vi "imp_2motor_v1.vi"() -> ()   [LabVIEW 2014]
uses:
  <vilib>/LabVIEW Targets/FPGA/cRIO/shared/nicrio_ModuleControls/nicrio_cRIO-9237_DataRatesRing.ctl
  <vilib>/LabVIEW Targets/FPGA/cRIO/shared/nicrio_ModuleControls/nicrio_cRIO-9237_ExcitationVoltageRing.ctl
  <vilib>/rvi/FXPMathLib/FxpSinAndCos/subVIs/nifxpmath_SinAndCos_SimConfig.ctl
  <vilib>/rvi/Emulation/niFpgaGetClockAttributes.vi
  <vilib>/rvi/Emulation/niFpgaSctlEmulationGetInTimedLoop.vi
  <vilib>/rvi/Emulation/niFpgaEmulationReportErrorSimple.vi
  <vilib>/rvi/Emulation/niFpgaProcessEmulError.vi
  <vilib>/rvi/interface/RandomDataEmulation/nirviRandomDataMultiElementFPGAFIFO.vi
  <instcachedir>/0/nirviRandomDataMultiElementFPGAFIFO_AD0CFC12EF974623A9C2E4184BC062B2.lvgen/nirviRandomDataMultiElementFPGAFIFO_AD0CFC12EF974623A9C2E4184BC062B2_023.vi
  <vilib>/rvi/interface/RandomDataEmulation/niFpgaRandomDataHandleErrors.vi
  <vilib>/rvi/Emulation/niFpgaCriticalErrorInLSC.vi
  <vilib>/rvi/eio/common/nirviEmuTemplateMethod_errors.vi
  <vilib>/rvi/FXPMathLib/FxpSinAndCos/simVIs/DllFxpSinAndCosTemp_sub.vi
  <vilib>/rvi/eio/common/nirviEmuTemplatePropertySet_errors.vi
  <vilib>/rvi/DataTransferAndStorage/Container/XNode/niFpgaContainer.xnode
  <vilib>/rvi/interface/RandomDataEmulation/nirviRandomDataFpgaMultiElementTemplate.vi
  <vilib>/eio/EIONode/EIONode.xnode
  <vilib>/rvi/FXPMathLib/FxpMul/XNode/nifxpmath_Multiplier.xnode
  <vilib>/rvi/FXPMathLib/FxpSinAndCos/XNode/nifxpmath_SinAndCos.xnode
  <vilib>/rvi/Analysis/measure/butterworth/XNode/niFpgaButterworthFilter.xnode
  <vilib>/rvi/FXPMathLib/FxpSub/XNode/nifxpmath_Sub.xnode
  <vilib>/rvi/FXPMathLib/FxpAdd/XNode/nifxpmath_Add.xnode
  <vilib>/eio/EIOPropertyNode/EIOPropertyNode.xnode
  <vilib>/rvi/eio/common/nirviEmuTemplatePropertyGet_errors.vi
  <vilib>/rvi/eio/common/nirviEmuTemplatePropertyGet_noerrors.vi
  <vilib>/rvi/eio/common/nirviEmuTemplatePropertySet_noerrors.vi
  <vilib>/rvi/FXPMathLib/sim/FxpSim.dll
panel:
  out "fpt_d":fxp<+/-,36,18>
  out "Dp_error_dd":fxp<+/-,36,16>
  out "Dp_error_d":fxp<+/-,33,8>
  in  "Dp_dd coeff.":i32[](array[numeric])=[946630756, 63555534]
  out "Dp_dd":fxp<+/-,36,25>
  out "dFp_PID":fxp<+/-,36,18>
  in  "dFp_PID coeff.":i32[](array[numeric])=[946630756, 63555534]
  out "fpt_i":fxp<+/-,34,18>
  in  "Bv_p":fxp<+/-,22,8>
  in  "Kv_p":fxp<+/-,22,8>
  out "Dp_error":fxp<+/-,22,7>
  out "Dpr_sin":fxp<+/-,22,7>
  in  "Sin offset_p":fxp<+/-,22,7>
  in  "Sin magnitude_p":fxp<+/-,21,6>
  out "Dpr_sin_dd":fxp<+/-,35,20>
  out "Dpr_sin_d":fxp<+/-,33,15>
  out "Sin omega_p":fxp<+/-,34,9>
  in  "Sin wave freq._p (Hz)":fxp<+/-,32,6>
  in  "Dpr_step":fxp<+/-,22,7>
  out "Dpr_for":fxp<+/-,22,7>
  in  "Command_p":i16(ring) items=["Step", "Sine"]
  in  "Ki_p":fxp<+/-,36,9>
  out "Fp_PID":fxp<+/-,36,16>
  in  "fp_tolorance":fxp<+,22,6>
  out "fp_tilde":fxp<+/-,33,10>
  in  "Kd_p":fxp<+/-,36,9>
  in  "Kp_p":fxp<+/-,36,9>
  out "Fr_p":fxp<+/-,32,10>
  in  "S/F coeff_p":fxp<+/-,25,-10>
  in  "S/F coeff_y":fxp<+/-,25,-10>
  out "va_p":fxp<+/-,36,7>
  out "vb_p":fxp<+/-,37,8>
  out "vq_p_F":fxp<+/-,20,5> format="%.57g"
  out "vd_p_F":fxp<+/-,20,5>
  in  "dFp_add":bool
  in  "Stop motor_p":bool
  out "Force_p":fxp<+/-,32,10>
  in  "Strain selection_p":i16(ring) items=["Raw", "Avg.", "Avg. w. filter"]
  out "Strain_p (Avg w. f)":fxp<+/-,36,8>
  in  "Strain_p mean coeff.":i32[](array[numeric])=[946630756, 63555534]
  out "Strain_p (Avg)":fxp<+/-,32,4>
  out "Raw Strain_p":fxp<+/-,36,4>
  out "Mod6/AI3":fxp<+/-,32,4>
  in  "Strain gage reset_p":bool
  out "Dp_d (mm/s)":fxp<+/-,36,11>
  out "omega_p (rad/s)":fxp<+/-,20,9>
  out "mt_omega_p":u32
  out "rad_p(NrTheta)":fxp<+/-,33,20>
  out "D_p(mm)":fxp<+/-,32,7>
  out "Encoder Position_p":i32
  in  "Encoder reset_p":bool
  out "Strain_y (Avg w. f)":fxp<+/-,36,8>
  in  "Strain_y mean coeff.":i32[](array[numeric])=[-898916953, 1957103773, 3888751]
  out "Dyr_for":fxp<+/-,22,7>
  in  "Command_y":i16(ring) items=["Step", "Sine"]
  out "Strain_y (Avg)":fxp<+/-,32,4>
  in  "Strain selection_y":i16(ring) items=["Raw", "Avg.", "Avg. w. filter"]
  out "vb_y":fxp<+/-,38,8>
  out "va_y":fxp<+/-,38,8>
  out "fyt_d":fxp<+/-,36,18>
  out "Fr_y":fxp<+/-,32,10>
  in  "Bv_y":fxp<+/-,22,8>
  out "Dy_error_dd":fxp<+/-,36,16>
  out "Dy_error_d":fxp<+/-,33,8>
  in  "Kv_y":fxp<+/-,22,8>
  out "Dy_error":fxp<+/-,22,7>
  out "Dyr_sin_dd":fxp<+/-,35,20>
  out "Dyr_sin_d":fxp<+/-,33,15>
  out "Sin omega_y":fxp<+/-,34,9>
  out "Dyr_sin":fxp<+/-,22,7>
  in  "Sin offset_y":fxp<+/-,22,7>
  in  "Sin magnitude_y":fxp<+/-,21,6>
  out "Time now(s)":fxp<+,52,14>
  in  "Sin wave freq._y (Hz)":fxp<+/-,32,6>
  in  "Dyr_step":fxp<+/-,22,7>
  in  "Drive mode":i16(ring) items=["Backward", "Forward"]
  out "Dy_dd":fxp<+/-,36,25>
  in  "Dy_dd coeff.":i32[](array[numeric])=[946630756, 63555534]
  out "dFy_PID":fxp<+/-,36,18>
  in  "dFy_PID coeff.":i32[](array[numeric])=[946630756, 63555534]
  out "fyt_i":fxp<+/-,36,16>
  out "Fy_PID":fxp<+/-,36,16>
  in  "fy_tolorance":fxp<+,22,6>
  in  "Ki_y":fxp<+/-,36,9>
  in  "Kd_y":fxp<+/-,36,9>
  out "fy_tilde":fxp<+/-,32,10>
  in  "Kp_y":fxp<+/-,36,9>
  out "vq_y_F":fxp<+/-,20,5> format="%.57g"
  out "vd_y_F":fxp<+/-,20,5>
  in  "dFy_add":bool
  in  "Stop motor_y":bool
  out "Dy_d (mm/s)":fxp<+/-,36,11>
  out "omega_y (rad/s)":fxp<+/-,20,9>
  in  "mt0_omega":u32
  out "mt_omega_y":u32
  out "rad_y(NrTheta)":fxp<+/-,33,20>
  out "D_y(mm)":fxp<+/-,32,7>
  out "Encoder Position_y":i32
  in  "Encoder reset_y":bool
  in  "Ini coe.":bool
  out "Loop rate_y (kHz)":fxp<+/-,36,7>
  out "Force_y":fxp<+/-,32,10>
  out "Raw Strain_y":fxp<+/-,36,4>
  in  "Strain gage reset_y":bool
  in  "Stop (Strain)":bool
  out "Mod6/AI2":fxp<+/-,32,4>
  in  "Excitation Voltage":T1 items=["2.5 Volts", "3.3 Volts", "5.0 Volts", "10.0 Volts", "External Excitation"]
  in  "Data Rate":T2=1 items=["50.000 kS/s (NI 9237)"=1, "25.000 kS/s (NI 9237)"=2, "16.667 kS/s (NI 9237)"=3, "12.500 kS/s (NI 9237)"=4, "10.000 kS/s (NI 9237)"=5, "8.333 kS/s (NI 9237)"=6, "7.143 kS/s (NI 9237)"=7, "6.250 kS/s (NI 9237)"=8, "5.556 kS/s (NI 9237)"=9, "5.000 kS/s (NI 9237)"=10, "4.545 kS/s (NI 9237)"=11, "4.167 kS/s (NI 9237)"=12, "3.846 kS/s (NI 9237)"=13, "3.571 kS/s (NI 9237)"=14, "3.333 kS/s (NI 9237)"=15, "3.125 kS/s (NI 9237)"=16, "2.941 kS/s (NI 9237)"=17, "2.778 kS/s (NI 9237)"=18, "2.632 kS/s (NI 9237)"=19, "2.500 kS/s (NI 9237)"=20, "2.381 kS/s (NI 9237)"=21, "2.273 kS/s (NI 9237)"=22, "2.174 kS/s (NI 9237)"=23, "2.083 kS/s (NI 9237)"=24, "2.000 kS/s (NI 9237)"=25, "1.923 kS/s (NI 9237)"=26, "1.852 kS/s (NI 9237)"=27, "1.786 kS/s (NI 9237)"=28, "1.724 kS/s (NI 9237)"=29, "1.667 kS/s (NI 9237)"=30, "1.613 kS/s (NI 9237)"=31]
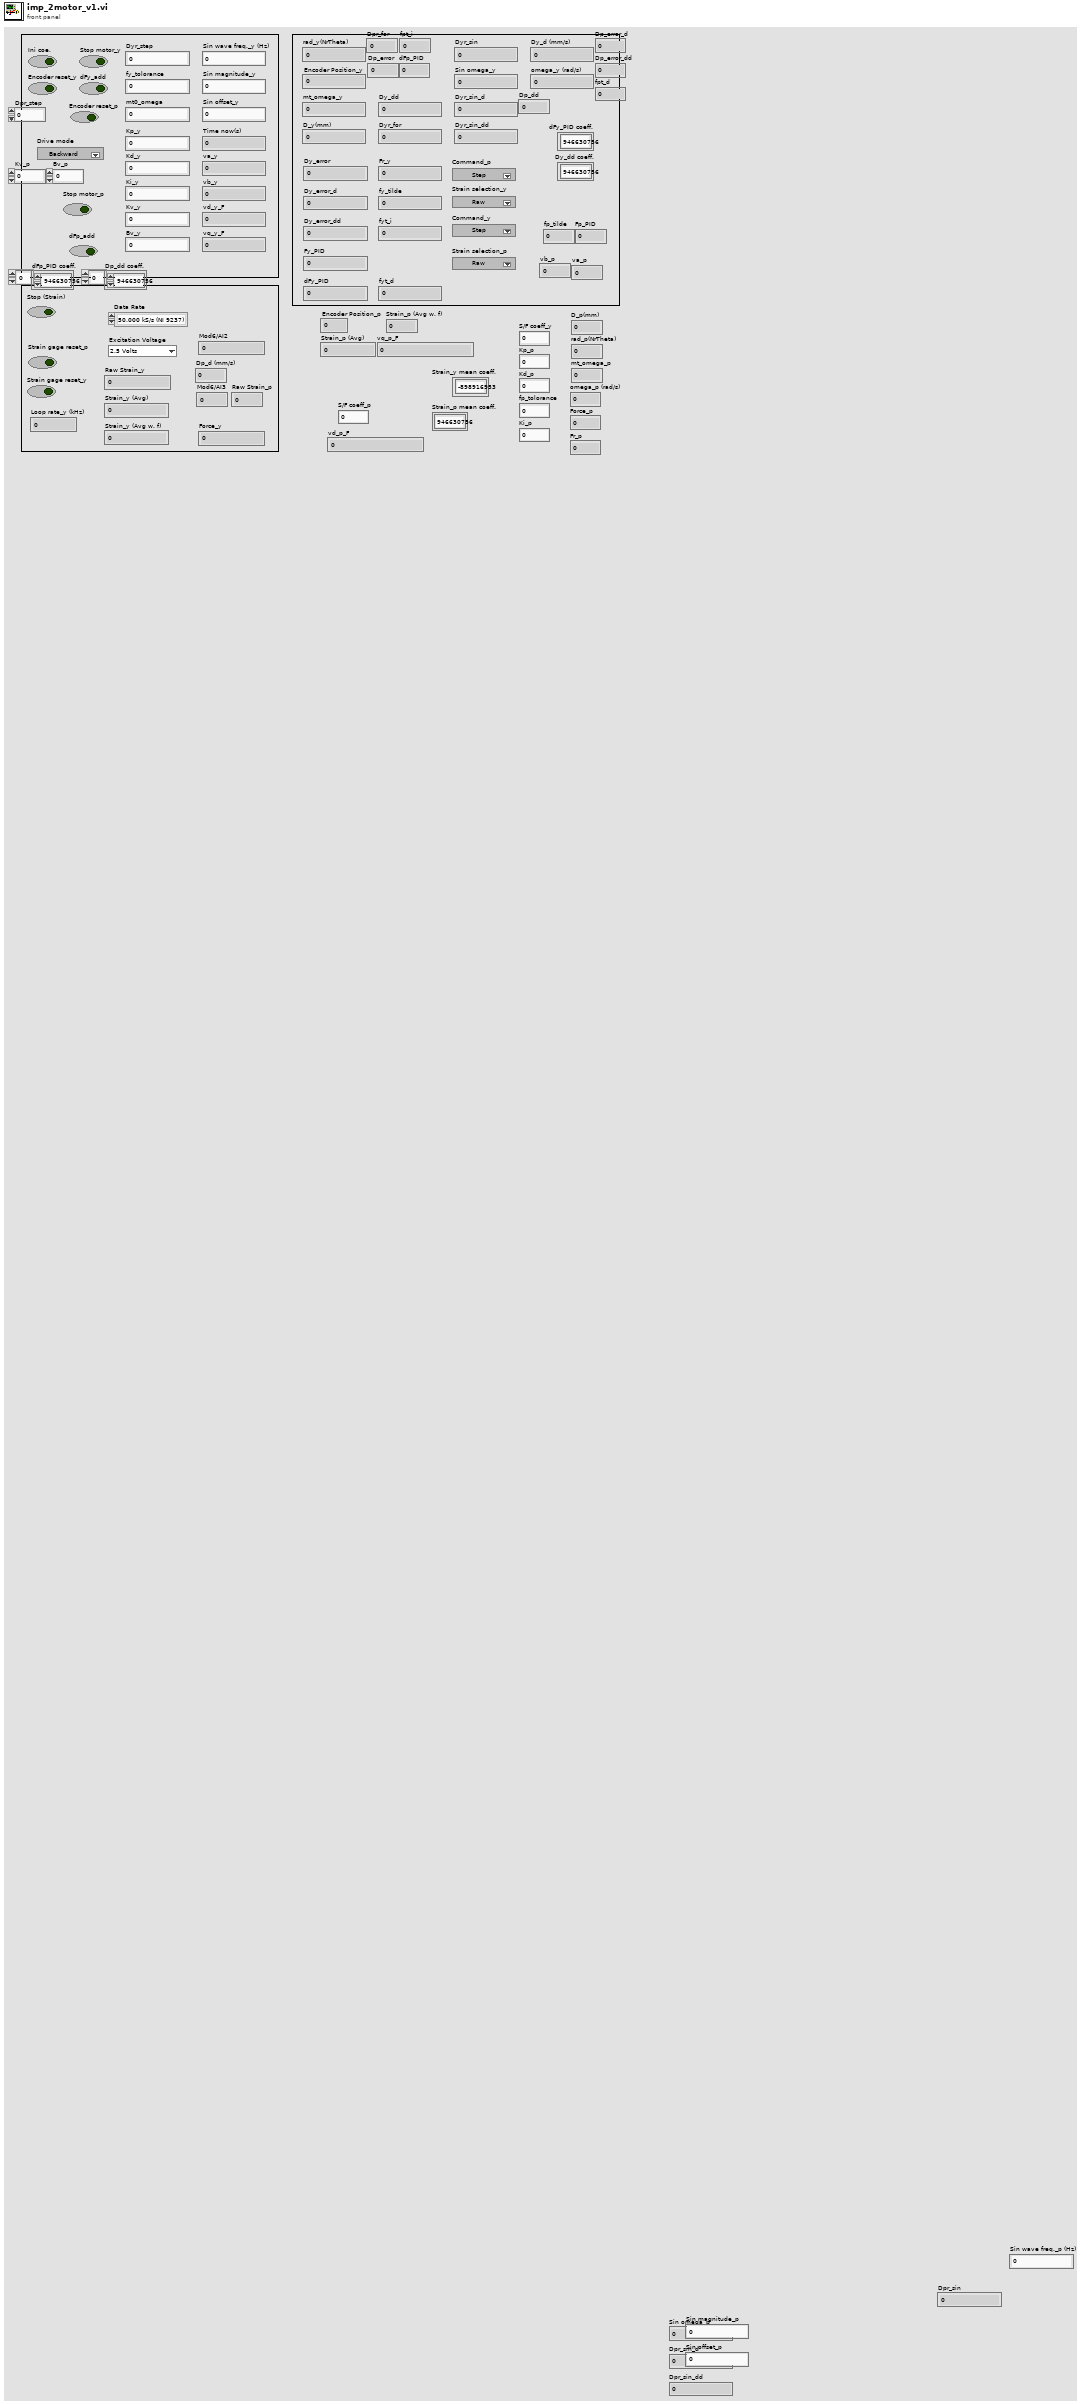
[diagram p1: front panel]
types:
  T1 = typedef "nicrio_cRIO-9237_ExcitationVoltageRing.ctl" = u8
  T2 = typedef "nicrio_cRIO-9237_DataRatesRing.ctl" = u8
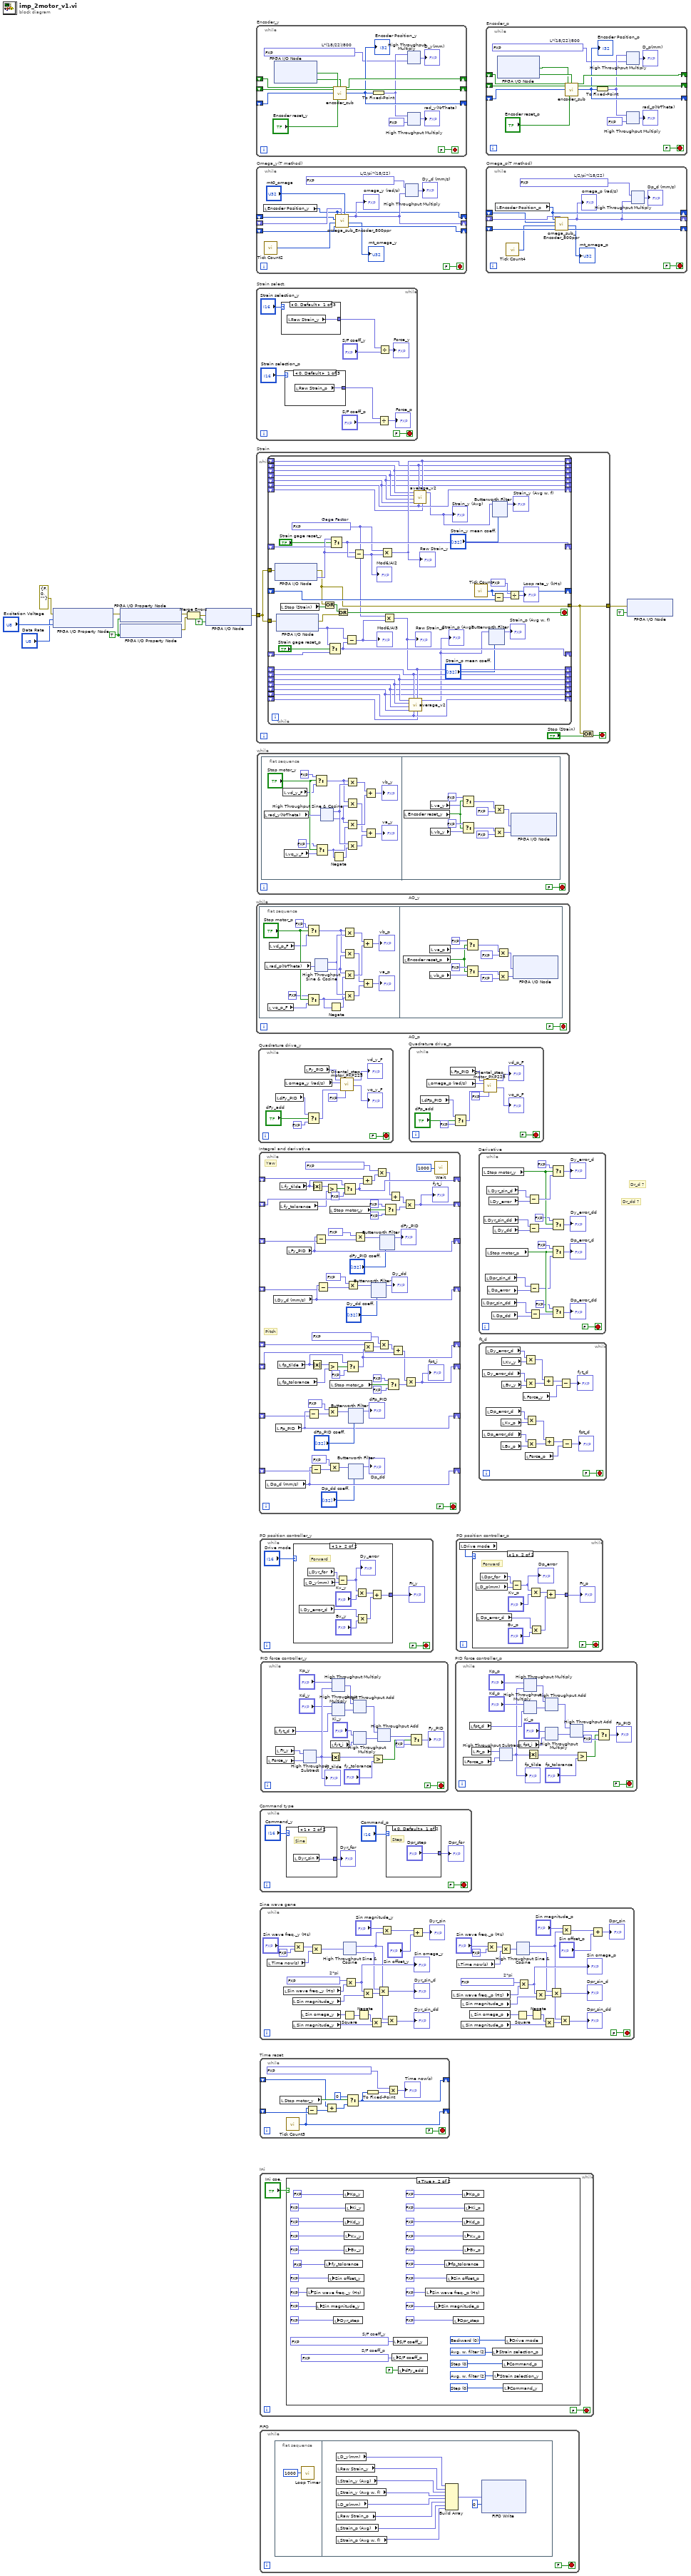
[diagram p0: block diagram]
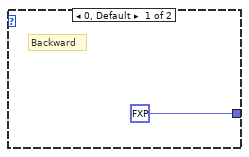
[diagram p2: hidden frame]
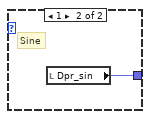
[diagram p3: hidden frame]
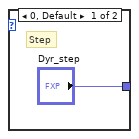
[diagram p4: hidden frame]
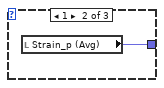
[diagram p5: hidden frame]
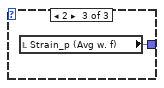
[diagram p6: hidden frame]
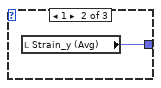
[diagram p7: hidden frame]
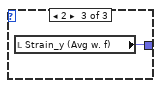
[diagram p8: hidden frame]
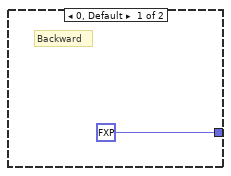
[diagram p9: hidden frame]
diagram:
  w5 = TRUE ("Half-Bridge Enable")
  # "Dr_dd ?"
  # "Dr_d ?"
  n1 = xnode "FPGA I/O Property Node"("error in"=errorcluster {"status"=FALSE, "code"=0, "source"=""}, "Data Rate"="Data Rate", "Excitation Voltage"="Excitation Voltage") -> ("error out"=w10:errorcluster)  [unwired: 1 in, 1 out]
  n2 = xnode "FPGA I/O Property Node"("error in"=w10, "Half-Bridge Enable"=w5) -> ("error out"=w3:errorcluster)  [unwired: 1 in, 1 out]
  n3 = xnode "FPGA I/O Property Node"("Half-Bridge Enable"=w5) -> ("error out"=w2:errorcluster)  [unwired: 2 in, 1 out]
  n4 = Merge Errors(w3, w2) -> (w4:errorcluster)
  n5 = xnode "FPGA I/O Node"("error in"=w4, "Mod6/Start"=TRUE) -> ("error out"=w8:errorcluster)  [unwired: 1 in, 1 out]
  n6 = while "Encoder_y" {
    shift-right: [w24] -> _
    shift-left: _ -> [w25]
    shift-right: [w26] -> _
    shift-left: _ -> [w27]
    shift-right: [w19] -> _
    shift-left: _ -> [w23]
    stop <- FALSE stop-if-true
    w16 = fxp<+/-,32,0> 0.0020454544574022293  # L*(18/22)/800
    n7 = xnode "FPGA I/O Node"() -> ("Mod4/DI3"=w22:bool, "Mod4/DI4"=w21:bool)  [unwired: 2 in, 2 out]
    n8 = call "encoder_sub.vi"("A_pre"=w25, "B_pre"=w27, "Encoder Position_pre"=w23, "A input"=w22, "Encoder Position Reset"="Encoder reset_y", "B input"=w21) -> ("A"=w24:bool, "B"=w26:bool, "Encoder Position (Counts)"=w19:i32)  [unwired: 19 in]
    "Encoder Position_y" <- w19
    n9 = To Fixed-Point(number=w19) -> (fixed-point=w18:fxp<+/-,32,32>)  [unwired: 1 in]
    n10 = xnode ("High Throughput Multiply")("x"=w18, "y"=w16) -> ("x*y"=→"D_y(mm)":fxp<+/-,64,32>)
    n11 = xnode ("High Throughput Multiply")("x"=w18, "y"=fxp<+/-,16,1> 0.125) -> ("x*y"=→"rad_y(NrTheta)":fxp<+/-,48,33>)
  }
  n12 = while "Omega_y(T method)" {
    shift-right: [w29] -> _
    shift-left: _ -> [w30]
    shift-right: [w33] -> _
    shift-left: _ -> [w35]
    shift-right: [w37] -> _
    shift-left: _ -> [w38]
    stop <- FALSE stop-if-true
    w32 = fxp<+/-,32,0> 0.2604353614151478  # L/2/pi*(18/22)
    n13 = local read "Encoder Position_y"() -> (w29:i32)
    n14 = call "Tick Count2"() -> ("Tick Count(Ticks)"=w39:u32)
    n15 = call "omega_sub_Encoder_800ppr.vi"("mt0"="mt0_omega", "omega_pre"=w35, "ticks_m_pre"=w38, "ticks"=w39, "count_pre"=w30, "count"=w29) -> ("ticks_m"=w37:u32, "mt"=→"mt_omega_y":u32, "omega"=w33:fxp<+/-,20,9>)  [unwired: 3 in]
    "omega_y (rad/s)" <- w33
    n16 = xnode ("High Throughput Multiply")("x"=w32, "y"=w33) -> ("x*y"=→"Dy_d (mm/s)":fxp<+/-,52,9>)
  }
  n17 = while "Strain select." {
    stop <- FALSE stop-if-true
    n18 = case shown="0, Default" "Strain selection_y" {
      tunnel: [w52 w53 w54] -> w46
      frame 0, Default {
        n19 = local read "Raw Strain_y"() -> (w52:fxp<+/-,36,4>)
      }
      frame 1 {
        n20 = local read "Strain_y (Avg)"() -> (w53:fxp<+/-,32,4>)
      }
      frame 2 {
        n21 = local read "Strain_y (Avg w. f)"() -> (w54:fxp<+/-,36,8>)
      }
    }
    n22 = case shown="0, Default" "Strain selection_p" {
      tunnel: [w49 w50 w51] -> w44
      frame 0, Default {
        n23 = local read "Raw Strain_p"() -> (w49:fxp<+/-,36,4>)
      }
      frame 1 {
        n24 = local read "Strain_p (Avg)"() -> (w50:fxp<+/-,32,4>)
      }
      frame 2 {
        n25 = local read "Strain_p (Avg w. f)"() -> (w51:fxp<+/-,36,8>)
      }
    }
    n26 = Divide(x=w44, y="S/F coeff_p") -> (x/y=→"Force_p":fxp<+/-,32,10>)
    n27 = Divide(x=w46, y="S/F coeff_y") -> (x/y=→"Force_y":fxp<+/-,32,10>)
  }
  n28 = while "Strain" {
    tunnel: w8 -> [w57]
    tunnel: [w55] -> w1
    stop <- w56 stop-if-true
    n29 = while {
      tunnel: w57 -> [w103]
      tunnel: [w76] -> w55
      shift-right: [w100] -> _
      shift-left: _ -> [w101]
      shift-right: [w96] -> _
      shift-left: _ -> [w97]
      shift-right: [w91] -> _
      shift-left: _ -> [w90]
      shift-right: [w90] -> _
      shift-left: _ -> [w89]
      shift-right: [w89] -> _
      shift-left: _ -> [w88]
      shift-right: [w88] -> _
      shift-left: _ -> [w87]
      shift-right: [w87] -> _
      shift-left: _ -> [w86]
      shift-right: [w86] -> _
      shift-left: _ -> [w85]
      shift-right: [w85] -> _
      shift-left: _ -> [w84]
      tunnel: w57 -> [w80]
      shift-right: [w73] -> _
      shift-left: _ -> [w74]
      shift-right: [w69] -> _
      shift-left: _ -> [w68]
      shift-right: [w68] -> _
      shift-left: _ -> [w67]
      shift-right: [w67] -> _
      shift-left: _ -> [w66]
      shift-right: [w66] -> _
      shift-left: _ -> [w65]
      shift-right: [w65] -> _
      shift-left: _ -> [w64]
      shift-right: [w64] -> _
      shift-left: _ -> [w63]
      shift-right: [w63] -> _
      shift-left: _ -> [w62]
      stop <- w77 stop-if-true
      w71 = fxp<+,20,2> 2.115001678466797  # Gage Factor
      n30 = xnode "FPGA I/O Node"("error in"=w103) -> ("error out"=w76:errorcluster, "Mod6/AI2"=w98:fxp<+/-,24,-4>)  [unwired: 1 in, 1 out]
      n31 = xnode "FPGA I/O Node"("error in"=w80) -> ("error out"=w78:errorcluster, "Mod6/AI3"=w72:fxp<+/-,24,-4>)  [unwired: 1 in, 1 out]
      n32 = local read "Stop (Strain)"() -> (w102:bool)
      n33 = Or(x=w76, y=w102) -> (x .or. y?=w79:bool)
      n34 = Select(t=w72, s="Strain gage reset_p", f=w74) -> (s? t:f=w73:fxp<+/-,24,-4>)
      n35 = Select(t=w98, s="Strain gage reset_y", f=w101) -> (s? t:f=w100:fxp<+/-,24,-4>)
      n36 = Or(x=w79, y=w78) -> (x .or. y?=w77:bool)
      n37 = Subtract(x=w72, y=w73) -> (x-y=w70:fxp<+/-,25,-3>)
      "Mod6/AI3" <- w70
      n38 = Subtract(x=w98, y=w100) -> (x-y=w99:fxp<+/-,25,-3>)
      "Mod6/AI2" <- w99
      n39 = Multiply(x=w71, y=w99) -> (x*y=w91:fxp<+/-,41,6>)
      "Raw Strain_y" <- w91
      n40 = Multiply(x=w71, y=w70) -> (x*y=w69:fxp<+/-,45,-1>)
      "Raw Strain_p" <- w69
      n41 = call "average_v2.vi"("Numeric 8"=w62, "Numeric"=w69, "Numeric 7"=w63, "Numeric 2"=w68, "Numeric 6"=w64, "Numeric 5"=w65, "Numeric 4"=w66, "Numeric 3"=w67) -> ("mean"=w61:fxp<+/-,32,4>)  [unwired: 2 in, 1 out]
      "Strain_p (Avg)" <- w61
      n42 = call "average_v2.vi"("Numeric 8"=w84, "Numeric"=w91, "Numeric 7"=w85, "Numeric 2"=w90, "Numeric 6"=w86, "Numeric 5"=w87, "Numeric 4"=w88, "Numeric 3"=w89) -> ("mean"=w83:fxp<+/-,32,4>)  [unwired: 2 in, 1 out]
      "Strain_y (Avg)" <- w83
      n43 = call "Tick Count"() -> ("Tick Count(uSec)"=w96:u32)
      n44 = xnode "Butterworth Filter"("input data"=w61, "scaled coefficients"="Strain_p mean coeff.") -> ("output data"=→"Strain_p (Avg w. f)":fxp<+/-,36,8>)  [unwired: 1 in]
      n45 = xnode "Butterworth Filter"("input data"=w83, "scaled coefficients"="Strain_y mean coeff.") -> ("output data"=→"Strain_y (Avg w. f)":fxp<+/-,32,4>)  [unwired: 1 in]
      n46 = Subtract(x=w96, y=w97) -> (x-y=w94:fxp<+/-,32,16>)
      n47 = Divide(x=fxp<+,7,10> 1000.0, y=w94) -> (x/y=→"Loop rate_y (kHz)":fxp<+/-,40,27>)
    }
    n48 = Or(x=w55, y="Stop (Strain)") -> (x .or. y?=w56:bool)
  }
  n49 = while "AO_p" {
    stop <- FALSE stop-if-true
    n50 = flat-sequence {
      frame #0 {
        n51 = local read "rad_p(NrTheta)"() -> (w132:fxp<+/-,33,20>)
        n52 = local read "vq_p_F"() -> (w133:fxp<+/-,20,5>)
        n53 = local read "vd_p_F"() -> (w135:fxp<+/-,20,5>)
        n54 = Select(t=fxp<+/-,20,5> 0.0, s="Stop motor_p", f=w135) -> (s? t:f=w124:fxp<+/-,20,5>)
        n55 = Select(t=fxp<+,1,1> 0.0, s="Stop motor_p", f=w133) -> (s? t:f=w123:fxp<+/-,20,5>)
        n56 = xnode "High Throughput Sine & Cosine"("x (pi)"=w132) -> ("sin(x)"=w126:fxp<+/-,16,2>, "cos(x)"=w125:fxp<+/-,16,2>)
        n57 = Negate(x=w123) -> (-x=w131:fxp<+/-,21,6>)
        n58 = Multiply(x=w124, y=w126) -> (x*y=w130:fxp<+/-,36,7>)
        n59 = Multiply(x=w124, y=w125) -> (x*y=w128:fxp<+/-,36,7>)
        n60 = Multiply(x=w125, y=w123) -> (x*y=w129:fxp<+/-,36,7>)
        n61 = Multiply(x=w126, y=w131) -> (x*y=w127:fxp<+/-,35,6>)
        n62 = Add(x=w130, y=w129) -> (x+y=→"vb_p":fxp<+/-,37,8>)
        n63 = Add(x=w128, y=w127) -> (x+y=→"va_p":fxp<+/-,36,7>)
      }
      frame #1 {
        n64 = local read "Encoder reset_p"() -> (w168:bool)
        n65 = local read "vb_p"() -> (w169:fxp<+/-,37,8>)
        n66 = local read "va_p"() -> (w170:fxp<+/-,36,7>)
        n67 = Select(t=fxp<+,2,2> 3.0, s=w168, f=w170) -> (s? t:f=w176:fxp<+/-,36,7>)
        n68 = Select(t=fxp<+,1,1> 0.0, s=w168, f=w169) -> (s? t:f=w175:fxp<+/-,37,8>)
        n69 = Multiply(x=w176, y=fxp<+/-,1,0> -0.5) -> (x*y=w171:fxp<+/-,36,6>)
        n70 = Multiply(x=w175, y=fxp<+/-,1,0> -0.5) -> (x*y=w172:fxp<+/-,36,6>)
        n71 = xnode "FPGA I/O Node"("Mod8/AO0"=w171, "Mod8/AO1"=w172) -> ()  [unwired: 2 in, 2 out]
      }
    }
  }
  n72 = while "AO_y" {
    stop <- FALSE stop-if-true
    n73 = flat-sequence {
      frame #0 {
        n74 = local read "rad_y(NrTheta)"() -> (w196:fxp<+/-,33,20>)
        n75 = local read "vd_y_F"() -> (w194:fxp<+/-,20,5>)
        n76 = local read "vq_y_F"() -> (w193:fxp<+/-,20,5>)
        n77 = Select(t=fxp<+/-,20,5> 0.0, s="Stop motor_y", f=w194) -> (s? t:f=w188:fxp<+/-,20,5>)
        n78 = Select(t=fxp<+/-,20,5> 0.0, s="Stop motor_y", f=w193) -> (s? t:f=w187:fxp<+/-,20,5>)
        n79 = xnode "High Throughput Sine & Cosine"("x (pi)"=w196) -> ("sin(x)"=w190:fxp<+/-,17,2>, "cos(x)"=w189:fxp<+/-,17,2>)
        n80 = Negate(x=w187) -> (-x=w186:fxp<+/-,21,6>)
        n81 = Multiply(x=w188, y=w190) -> (x*y=w185:fxp<+/-,37,7>)
        n82 = Multiply(x=w188, y=w189) -> (x*y=w183:fxp<+/-,37,7>)
        n83 = Multiply(x=w189, y=w187) -> (x*y=w184:fxp<+/-,37,7>)
        n84 = Multiply(x=w190, y=w186) -> (x*y=w182:fxp<+/-,36,6>)
        n85 = Add(x=w185, y=w184) -> (x+y=→"vb_y":fxp<+/-,38,8>)
        n86 = Add(x=w183, y=w182) -> (x+y=→"va_y":fxp<+/-,37,7>)
      }
      frame #1 {
        n87 = local read "Encoder reset_y"() -> (w229:bool)
        n88 = local read "va_y"() -> (w228:fxp<+/-,38,8>)
        n89 = local read "vb_y"() -> (w227:fxp<+/-,38,8>)
        n90 = Select(t=fxp<+,2,2> 3.0, s=w229, f=w228) -> (s? t:f=w233:fxp<+/-,38,8>)
        n91 = Select(t=fxp<+,1,1> 0.0, s=w229, f=w227) -> (s? t:f=w232:fxp<+/-,38,8>)
        n92 = Multiply(x=w233, y=fxp<+/-,1,0> -0.5) -> (x*y=w236:fxp<+/-,39,8>)
        n93 = Multiply(x=w232, y=fxp<+/-,1,0> -0.5) -> (x*y=w237:fxp<+/-,37,6>)
        n94 = xnode "FPGA I/O Node"("Mod8/AO2"=w236, "Mod8/AO3"=w237) -> ()  [unwired: 2 in, 2 out]
      }
    }
  }
  n95 = while "Quadrature drive_y" {
    stop <- FALSE stop-if-true
    n96 = local read "dFy_PID"() -> (w239:fxp<+/-,36,18>)
    n97 = local read "omega_y (rad/s)"() -> (w247:fxp<+/-,20,9>)
    n98 = local read "Fy_PID"() -> (w240:fxp<+/-,36,16>)
    n99 = Select(t=w239, s="dFy_add", f=fxp<+,1,1> 0.0) -> (s? t:f=w243:fxp<+/-,36,18>)
    n100 = call "Oriental_step_motor_PKP225.vi"("F_Threshold"=fxp<+,12,12> 10.0, "dFmr"=w243, "omega"=w247, "Fmr"=w240) -> ("vq_F"=→"vq_y_F":fxp<+/-,20,5>, "vd_F"=→"vd_y_F":fxp<+/-,20,5>)  [unwired: 6 in]
  }
  n101 = while "Integral and derivative" {
    shift-right: [w303] -> _
    shift-left: _ -> [w302]
    shift-right: [w295] -> _
    shift-left: _ -> [w294]
    shift-right: [w305] -> _
    shift-left: _ -> [w306]
    shift-right: [w285] -> _
    shift-left: _ -> [w284]
    shift-right: [w271] -> _
    shift-left: _ -> [w274]
    shift-right: [w264] -> _
    shift-left: _ -> [w263]
    shift-right: [w258] -> _
    shift-left: _ -> [w257]
    shift-right: [w253] -> _
    shift-left: _ -> [w254]
    stop <- FALSE stop-if-true
    # "Pitch"
    # "Yaw"
    n102 = local read "Dp_d (mm/s)"() -> (w253:fxp<+/-,36,11>)
    n103 = local read "Dy_d (mm/s)"() -> (w285:fxp<+/-,36,11>)
    n104 = local read "Fp_PID"() -> (w258:fxp<+/-,36,16>)
    n105 = local read "fp_tilde"() -> (w275:fxp<+/-,33,10>)
    n106 = local read "fp_tolorance"() -> (w278:fxp<+,22,6>)
    n107 = local read "fy_tolorance"() -> (w281:fxp<+,22,6>)
    n108 = local read "fy_tilde"() -> (w307:fxp<+/-,32,10>)
    n109 = local read "Fy_PID"() -> (w305:fxp<+/-,36,16>)
    n110 = Subtract(x=w258, y=w257) -> (x-y=w262:fxp<+/-,37,17>)
    n111 = Subtract(x=w253, y=w254) -> (x-y=w255:fxp<+/-,37,12>)
    n112 = Absolute Value(x=w275) -> (abs(x)=w279:fxp<+,33,10>)
    n113 = Absolute Value(x=w307) -> (abs(x)=w309:fxp<+,32,10>)
    n114 = Subtract(x=w305, y=w306) -> (x-y=w293:fxp<+/-,37,17>)
    n115 = Subtract(x=w285, y=w284) -> (x-y=w287:fxp<+/-,36,11>)
    n116 = Greater?(x=w309, y=w281) -> (0:w310:bool)
    n117 = Greater?(x=w279, y=w278) -> (0:w277:bool)
    n118 = Multiply(x=fxp<+,7,10> 1000.0, y=w262) -> (x*y=w260:fxp<+/-,32,18>)
    n119 = Multiply(x=fxp<+,7,10> 1000.0, y=w255) -> (x*y=w251:fxp<+/-,36,21>)
    n120 = local read "Stop motor_y"() -> (w296:bool)
    n121 = local read "Stop motor_p"() -> (w266:bool)
    n122 = Select(t=w307, s=w310, f=fxp<+/-,33,11> 0.0) -> (s? t:f=w303:fxp<+/-,33,11>)
    n123 = Select(t=w275, s=w277, f=fxp<+,1,1> 0.0) -> (s? t:f=w271:fxp<+/-,33,10>)
    n124 = Multiply(x=fxp<+,7,10> 1000.0, y=w287) -> (x*y=w286:fxp<+/-,36,21>)
    n125 = xnode "Butterworth Filter"("input data"=w260, "scaled coefficients"="dFp_PID coeff.") -> ("output data"=→"dFp_PID":fxp<+/-,36,22>)  [unwired: 1 in]
    n126 = xnode "Butterworth Filter"("input data"=w251, "scaled coefficients"="Dp_dd coeff.") -> ("output data"=→"Dp_dd":fxp<+/-,36,25>)  [unwired: 1 in]
    n127 = Multiply(x=fxp<+,7,10> 1000.0, y=w293) -> (x*y=w290:fxp<+/-,32,18>)
    n128 = Add(x=w302, y=w303) -> (x+y=w308:fxp<+/-,34,12>)
    n129 = Multiply(x=w274, y=w271) -> (x*y=w273:fxp<+/-,34,12>)
    n130 = xnode "Butterworth Filter"("input data"=w286, "scaled coefficients"="Dy_dd coeff.") -> ("output data"=→"Dy_dd":fxp<+/-,36,25>)  [unwired: 1 in]
    n131 = Multiply(x=fxp<+/-,30,12> 0.000499725341796875, y=w308) -> (x*y=w301:fxp<+/-,34,10>)
    n132 = Multiply(x=fxp<+/-,30,12> 0.000499725341796875, y=w273) -> (x*y=w270:fxp<+/-,34,10>)
    n133 = xnode "Butterworth Filter"("input data"=w290, "scaled coefficients"="dFy_PID coeff.") -> ("output data"=→"dFy_PID":fxp<+/-,36,22>)  [unwired: 1 in]
    n134 = Select(t=fxp<+,1,1> 0.0, s=w296, f=fxp<+,1,1> 1.0) -> (s? t:f=w299:fxp<+,1,1>)
    n135 = Select(t=fxp<+,1,1> 0.0, s=w266, f=fxp<+,1,1> 1.0) -> (s? t:f=w268:fxp<+,1,1>)
    n136 = Add(x=w301, y=w294) -> (x+y=w300:fxp<+/-,36,16>)
    n137 = Add(x=w270, y=w263) -> (x+y=w269:fxp<+/-,36,16>)
    n138 = Multiply(x=w300, y=w299) -> (x*y=w295:fxp<+/-,34,18>)
    "fyt_i" <- w295
    n139 = Multiply(x=w269, y=w268) -> (x*y=w264:fxp<+/-,34,18>)
    "fpt_i" <- w264
    n140 = call "Wait"("Count(uSec)"=u32 1000) -> ()  [unwired: 1 out]
  }
  n141 = while "PD position controller_y" {
    stop <- FALSE stop-if-true
    n142 = case shown="1" "Drive mode" {
      tunnel: [fxp<+/-,62,19> 0.0 w349] -> w345
      frame 0, Default {
        # "Backward"
      }
      frame 1 {
        # "Forward"
        n143 = local read "Dy_error_d"() -> (w351:fxp<+/-,33,8>)
        n144 = local read "D_y(mm)"() -> (w356:fxp<+/-,32,7>)
        n145 = local read "Dyr_for"() -> (w348:fxp<+/-,22,7>)
        n146 = Subtract(x=w348, y=w356) -> (x-y=w355:fxp<+/-,33,8>)
        "Dy_error" <- w355
        n147 = Multiply(x=w355, y="Kv_y") -> (x*y=w353:fxp<+/-,54,15>)
        n148 = Multiply(x=w351, y="Bv_y") -> (x*y=w350:fxp<+/-,55,16>)
        n149 = Add(x=w353, y=w350) -> (x+y=w349:fxp<+/-,55,16>)
      }
    }
    "Fr_y" <- w345
  }
  n150 = while "Command type" {
    stop <- FALSE stop-if-true
    n151 = case shown="1" "Command_y" {
      tunnel: ["Dyr_step" w365] -> w360
      frame 0, Default {
        # "Step"
      }
      frame 1 {
        # "Sine"
        n152 = local read "Dyr_sin"() -> (w365:fxp<+/-,22,7>)
      }
    }
    "Dyr_for" <- w360
    n153 = case shown="0, Default" "Command_p" {
      tunnel: ["Dpr_step" w363] -> w358
      frame 0, Default {
        # "Step"
      }
      frame 1 {
        # "Sine"
        n154 = local read "Dpr_sin"() -> (w363:fxp<+/-,22,7>)
      }
    }
    "Dpr_for" <- w358
  }
  n155 = while "Sine wave gene" {
    stop <- FALSE stop-if-true
    w371 = fxp<+,20,3> 6.2831878662109375  # 2*pi
    w403 = fxp<+,20,3> 6.2831878662109375  # 2*pi
    n156 = local read "Time now(s)"() -> (w409:fxp<+,52,14>)
    n157 = local read "Sin wave freq._y (Hz)"() -> (w402:fxp<+/-,32,6>)
    n158 = Multiply(x="Sin wave freq._y (Hz)", y=fxp<+/-,10,3> 2.0) -> (x*y=w410:fxp<+/-,41,9>)
    n159 = local read "Sin magnitude_y"() -> (w400:fxp<+/-,21,6>)
    n160 = local read "Sin magnitude_y"() -> (w393:fxp<+/-,21,6>)
    n161 = local read "Sin omega_y"() -> (w396:fxp<+/-,34,9>)
    n162 = Multiply(x=w410, y=w409) -> (x*y=w408:fxp<+/-,41,19>)
    n163 = Square(x=w396) -> (x^2=w395:fxp<+,34,18>)
    n164 = xnode "High Throughput Sine & Cosine"("x (pi)"=w408) -> ("sin(x)"=w390:fxp<+/-,16,2>, "cos(x)"=w398:fxp<+/-,16,2>)
    n165 = Multiply(x=w403, y=w402) -> (x*y=w401:fxp<+/-,34,9>)
    "Sin omega_y" <- w401
    n166 = Negate(x=w395) -> (-x=w394:fxp<+/-,35,19>)
    n167 = Multiply(x=w401, y=w400) -> (x*y=w399:fxp<+/-,33,15>)
    n168 = Multiply(x=w394, y=w393) -> (x*y=w392:fxp<+/-,34,20>)
    n169 = Multiply(x=w398, y=w399) -> (x*y=→"Dyr_sin_d":fxp<+/-,33,15>)
    n170 = Multiply(x="Sin magnitude_y", y=w390) -> (x*y=w406:fxp<+/-,37,8>)
    n171 = Multiply(x=w390, y=w392) -> (x*y=→"Dyr_sin_dd":fxp<+/-,35,20>)
    n172 = Add(x=w406, y="Sin offset_y") -> (x+y=→"Dyr_sin":fxp<+/-,37,8>)
    n173 = local read "Sin wave freq._p (Hz)"() -> (w367:fxp<+/-,32,6>)
    n174 = local read "Time now(s)"() -> (w385:fxp<+,52,14>)
    n175 = local read "Sin magnitude_p"() -> (w368:fxp<+/-,21,6>)
    n176 = local read "Sin magnitude_p"() -> (w370:fxp<+/-,21,6>)
    n177 = local read "Sin omega_p"() -> (w369:fxp<+/-,34,9>)
    n178 = Multiply(x="Sin wave freq._p (Hz)", y=fxp<+/-,10,3> 2.0) -> (x*y=w389:fxp<+/-,42,9>)
    n179 = Multiply(x=w389, y=w385) -> (x*y=w386:fxp<+/-,41,19>)
    n180 = Square(x=w369) -> (x^2=w381:fxp<+,34,18>)
    n181 = xnode "High Throughput Sine & Cosine"("x (pi)"=w386) -> ("sin(x)"=w372:fxp<+/-,16,2>, "cos(x)"=w377:fxp<+/-,16,2>)
    n182 = Multiply(x=w371, y=w367) -> (x*y=w384:fxp<+/-,34,9>)
    "Sin omega_p" <- w384
    n183 = Negate(x=w381) -> (-x=w380:fxp<+/-,35,19>)
    n184 = Multiply(x=w384, y=w368) -> (x*y=w383:fxp<+/-,33,15>)
    n185 = Multiply(x=w380, y=w370) -> (x*y=w379:fxp<+/-,35,19>)
    n186 = Multiply(x=w377, y=w383) -> (x*y=→"Dpr_sin_d":fxp<+/-,33,15>)
    n187 = Multiply(x=w372, y=w379) -> (x*y=→"Dpr_sin_dd":fxp<+/-,35,20>)
    n188 = Multiply(x="Sin magnitude_p", y=w372) -> (x*y=w375:fxp<+/-,37,8>)
    n189 = Add(x=w375, y="Sin offset_p") -> (x+y=→"Dpr_sin":fxp<+/-,37,8>)
  }
  n190 = while "Time reset" {
    shift-right: [w482] -> _
    shift-left: _ -> [w483]
    shift-right: [w477] -> _
    shift-left: _ -> [w478]
    stop <- FALSE stop-if-true
    n191 = local read "Stop motor_y"() -> (w484:bool)
    n192 = call "Tick Count3"() -> ("Tick Count(uSec)"=w482:u32)
    n193 = Subtract(x=w482, y=w483) -> (x-y=w481:u32)
    n194 = Add(x=w478, y=w481) -> (x+y=w480:u32)
    n195 = Select(t=u32 0, s=w484, f=w480) -> (s? t:f=w477:u32)
    n196 = To Fixed-Point(number=w477) -> (fixed-point=w476:fxp<+,32,32>)  [unwired: 1 in]
    n197 = Multiply(x=fxp<+,20,-18> 1.0000003385357559e-06, y=w476) -> (x*y=→"Time now(s)":fxp<+,52,14>)
  }
  n198 = while "Ini" {
    stop <- FALSE stop-if-true
    n199 = case shown="True" "Ini coe." {
      frame False {
      }
      frame True {
        w497 = i16 0 items=["Step", "Sine"] ("Command_p")
        w498 = i16 2 items=["Raw", "Avg.", "Avg. w. filter"] ("Strain selection_p")
        w499 = i16 0 items=["Step", "Sine"] ("Command_y")
        w500 = i16 2 items=["Raw", "Avg.", "Avg. w. filter"] ("Strain selection_y")
        w502 = fxp<+/-,25,-10> 5.851034075021744e-07  # S/F coeff_p
        w501 = fxp<+/-,25,-10> -1.0477961041033268e-06  # S/F coeff_y
        w508 = i16 0 items=["Backward", "Forward"] ("Drive mode")
        n200 = local write "Sin wave freq._y (Hz)"(fxp<+/-,32,6> 1.0 ("Sin wave freq. (Hz)")) -> ()
        n201 = local write "Sin magnitude_y"(fxp<+/-,22,7> 5.0 ("Sin magnitude")) -> ()
        n202 = local write "fy_tolorance"(fxp<+,22,6> 10.0 ("f_tolorance")) -> ()
        n203 = local write "Sin offset_y"(fxp<+/-,38,9> 0.0 ("Sin offset")) -> ()
        n204 = local write "Dyr_step"(fxp<+/-,22,7> 0.0 ("Dr")) -> ()
        n205 = local write "Kp_y"(fxp<+/-,36,9> 30.0 ("Kp")) -> ()
        n206 = local write "Kd_y"(fxp<+/-,36,9> 0.0 ("Kd")) -> ()
        n207 = local write "Kv_y"(fxp<+/-,22,8> 0.0 ("Kv")) -> ()
        n208 = local write "Bv_y"(fxp<+/-,22,8> 0.0 ("Bv")) -> ()
        n209 = local write "Ki_y"(fxp<+/-,36,9> 0.0 ("Ki")) -> ()
        n210 = local write "S/F coeff_p"(w502) -> ()
        n211 = local write "S/F coeff_y"(w501) -> ()
        n212 = local write "dFy_add"(FALSE ("dF_add")) -> ()
        n213 = local write "Sin wave freq._p (Hz)"(fxp<+/-,32,6> 0.0 ("Sin wave freq._p (Hz)")) -> ()
        n214 = local write "Sin magnitude_p"(fxp<+/-,21,6> 0.0 ("Sin magnitude_p")) -> ()
        n215 = local write "fp_tolorance"(fxp<+,22,6> 0.0 ("fp_tolorance")) -> ()
        n216 = local write "Sin offset_p"(fxp<+/-,22,7> 0.0 ("Sin offset_p")) -> ()
        n217 = local write "Dpr_step"(fxp<+/-,22,7> 0.0 ("Dpr_step")) -> ()
        n218 = local write "Kp_p"(fxp<+/-,36,9> 0.0 ("Kp_p")) -> ()
        n219 = local write "Kd_p"(fxp<+/-,36,9> 0.0 ("Kd_p")) -> ()
        n220 = local write "Kv_p"(fxp<+/-,22,8> 0.0 ("Kv_p")) -> ()
        n221 = local write "Bv_p"(fxp<+/-,22,8> 0.0 ("Bv_p")) -> ()
        n222 = local write "Ki_p"(fxp<+/-,36,9> 0.0 ("Ki_p")) -> ()
        n223 = local write "Strain selection_p"(w498) -> ()
        n224 = local write "Strain selection_y"(w500) -> ()
        n225 = local write "Command_p"(w497) -> ()
        n226 = local write "Command_y"(w499) -> ()
        n227 = local write "Drive mode"(w508) -> ()
      }
    }
  }
  n228 = while "FIFO" {
    stop <- FALSE stop-if-true
    n229 = flat-sequence {
      frame #0 {
        n230 = call "Loop Timer"("Count(uSec)"=u32 1000) -> ()  [unwired: 1 out]
      }
      frame #1 {
        n231 = local read "D_y(mm)"() -> (w526:fxp<+/-,32,7>)
        n232 = local read "Raw Strain_y"() -> (w525:fxp<+/-,36,4>)
        n233 = local read "Strain_y (Avg)"() -> (w524:fxp<+/-,32,4>)
        n234 = local read "Strain_y (Avg w. f)"() -> (w523:fxp<+/-,36,8>)
        n235 = local read "D_p(mm)"() -> (w522:fxp<+/-,32,7>)
        n236 = local read "Raw Strain_p"() -> (w521:fxp<+/-,36,4>)
        n237 = local read "Strain_p (Avg)"() -> (w520:fxp<+/-,32,4>)
        n238 = local read "Strain_p (Avg w. f)"() -> (w517:fxp<+/-,36,8>)
        n239 = Build Array(w526, w525, w524, w523, w522, w521, w520, w517) -> (w519:fxp<+/-,40,8>[])
        n240 = xnode ("FIFO Write")("Element"=w519, "Timeout"=0) -> ()  [unwired: 1 in, 2 out]
      }
    }
  }
  n241 = while "PID force controller_y" {
    stop <- FALSE stop-if-true
    n242 = local read "Force_y"() -> (w544:fxp<+/-,32,10>)
    n243 = local read "fyt_d"() -> (w528:fxp<+/-,36,18>)
    n244 = local read "Fr_y"() -> (w530:fxp<+/-,32,10>)
    n245 = xnode "High Throughput Subtract"("x"=w530, "y"=w544) -> ("x-y"=w543:fxp<+/-,33,11>)
    "fy_tilde" <- w543
    n246 = Absolute Value(x=w543) -> (abs(x)=w534:fxp<+,33,11>)
    n247 = local read "fyt_i"() -> (w529:fxp<+/-,36,16>)
    n248 = xnode ("High Throughput Multiply")("x"="Kp_y", "y"=w543) -> ("x*y"=w541:fxp<+/-,64,20>)
    n249 = xnode ("High Throughput Multiply")("x"="Kd_y", "y"=w528) -> ("x*y"=w540:fxp<+/-,64,27>)
    n250 = xnode ("High Throughput Add")("x"=w541, "y"=w540) -> ("x+y"=w537:fxp<+/-,64,28>)
    n251 = xnode ("High Throughput Multiply")("x"="Ki_y", "y"=w529) -> ("x*y"=w538:fxp<+/-,64,25>)
    n252 = Greater?(x=w534, y="fy_tolorance") -> (0:w532:bool)
    n253 = xnode ("High Throughput Add")("x"=w537, "y"=w538) -> ("x+y"=w536:fxp<+/-,64,29>)
    n254 = Select(t=w536, s=w532, f=fxp<+/-,51,14> 0.0) -> (s? t:f=→"Fy_PID":fxp<+/-,64,29>)
  }
  n255 = while "Quadrature drive_p" {
    stop <- FALSE stop-if-true
    n256 = local read "dFp_PID"() -> (w547:fxp<+/-,36,18>)
    n257 = local read "omega_p (rad/s)"() -> (w553:fxp<+/-,20,9>)
    n258 = local read "Fp_PID"() -> (w548:fxp<+/-,36,16>)
    n259 = Select(t=w547, s="dFp_add", f=fxp<+,1,1> 0.0) -> (s? t:f=w551:fxp<+/-,36,18>)
    n260 = call "Oriental_step_motor_PKP225.vi"("F_Threshold"=fxp<+,12,12> 10.0, "dFmr"=w551, "omega"=w553, "Fmr"=w548) -> ("vq_F"=→"vq_p_F":fxp<+/-,20,5>, "vd_F"=→"vd_p_F":fxp<+/-,20,5>)  [unwired: 6 in]
  }
  n261 = while "PID force controller_p" {
    stop <- FALSE stop-if-true
    n262 = local read "Force_p"() -> (w568:fxp<+/-,32,10>)
    n263 = local read "fpt_d"() -> (w559:fxp<+/-,36,18>)
    n264 = local read "Fr_p"() -> (w569:fxp<+/-,32,10>)
    n265 = xnode "High Throughput Subtract"("x"=w569, "y"=w568) -> ("x-y"=w560:fxp<+/-,33,11>)
    "fp_tilde" <- w560
    n266 = local read "fpt_i"() -> (w557:fxp<+/-,34,18>)
    n267 = xnode "High Throughput Multiply"("x"="Kp_p", "y"=w560) -> ("x*y"=w558:fxp<+/-,64,20>)
    n268 = xnode "High Throughput Multiply"("x"="Kd_p", "y"=w559) -> ("x*y"=w574:fxp<+/-,64,27>)
    n269 = Absolute Value(x=w560) -> (abs(x)=w567:fxp<+,33,11>)
    n270 = xnode "High Throughput Add"("x"=w558, "y"=w574) -> ("x+y"=w572:fxp<+/-,64,28>)
    n271 = xnode "High Throughput Multiply"("x"="Ki_p", "y"=w557) -> ("x*y"=w573:fxp<+/-,64,27>)
    n272 = xnode "High Throughput Add"("x"=w572, "y"=w573) -> ("x+y"=w563:fxp<+/-,64,29>)
    n273 = Greater?(x=w567, y="fp_tolorance") -> (0:w564:bool)
    n274 = Select(t=w563, s=w564, f=fxp<+,1,1> 0.0) -> (s? t:f=→"Fp_PID":fxp<+/-,64,29>)
  }
  n275 = while "PD position controller_p" {
    stop <- FALSE stop-if-true
    n276 = local read "Drive mode"() -> (w577:i16)
    n277 = case shown="1" w577 {
      tunnel: [fxp<+/-,62,19> 0.0 w580] -> w576
      frame 0, Default {
        # "Backward"
      }
      frame 1 {
        # "Forward"
        n278 = local read "D_p(mm)"() -> (w587:fxp<+/-,32,7>)
        n279 = local read "Dp_error_d"() -> (w579:fxp<+/-,33,8>)
        n280 = local read "Dpr_for"() -> (w586:fxp<+/-,22,7>)
        n281 = Subtract(x=w586, y=w587) -> (x-y=w585:fxp<+/-,24,8>)
        "Dp_error" <- w585
        n282 = Multiply(x=w585, y="Kv_p") -> (x*y=w582:fxp<+/-,34,16>)
        n283 = Multiply(x=w579, y="Bv_p") -> (x*y=w581:fxp<+/-,55,16>)
        n284 = Add(x=w582, y=w581) -> (x+y=w580:fxp<+/-,56,17>)
      }
    }
    "Fr_p" <- w576
  }
  n285 = while "Derivative" {
    stop <- FALSE stop-if-true
    n286 = local read "Dpr_sin_dd"() -> (w596:fxp<+/-,35,20>)
    n287 = local read "Stop motor_y"() -> (w602:bool)
    n288 = local read "Dyr_sin_dd"() -> (w604:fxp<+/-,35,20>)
    n289 = local read "Dpr_sin_d"() -> (w598:fxp<+/-,33,15>)
    n290 = local read "Stop motor_p"() -> (w594:bool)
    n291 = local read "Dyr_sin_d"() -> (w607:fxp<+/-,33,15>)
    n292 = local read "Dp_error"() -> (w599:fxp<+/-,22,7>)
    n293 = local read "Dy_error"() -> (w608:fxp<+/-,22,7>)
    n294 = local read "Dp_dd"() -> (w597:fxp<+/-,36,25>)
    n295 = local read "Dy_dd"() -> (w605:fxp<+/-,36,25>)
    n296 = Subtract(x=w607, y=w608) -> (x-y=w606:fxp<+/-,34,16>)
    n297 = Subtract(x=w604, y=w605) -> (x-y=w603:fxp<+/-,41,26>)
    n298 = Subtract(x=w598, y=w599) -> (x-y=w591:fxp<+/-,34,16>)
    n299 = Subtract(x=w596, y=w597) -> (x-y=w595:fxp<+/-,41,26>)
    n300 = Select(t=fxp<+,1,1> 0.0, s=w602, f=w606) -> (s? t:f=→"Dy_error_d":fxp<+/-,34,16>)
    n301 = Select(t=fxp<+/-,64,49> 0.0, s=w602, f=w603) -> (s? t:f=→"Dy_error_dd":fxp<+/-,64,49>)
    n302 = Select(t=fxp<+,1,1> 0.0, s=w594, f=w591) -> (s? t:f=→"Dp_error_d":fxp<+/-,34,16>)
    n303 = Select(t=fxp<+/-,41,26> 0.0, s=w594, f=w595) -> (s? t:f=→"Dp_error_dd":fxp<+/-,41,26>)
  }
  n304 = while "ft_d" {
    stop <- FALSE stop-if-true
    n305 = local read "Dy_error_dd"() -> (w626:fxp<+/-,36,16>)
    n306 = local read "Dp_error_dd"() -> (w617:fxp<+/-,36,16>)
    n307 = local read "Dy_error_d"() -> (w628:fxp<+/-,33,8>)
    n308 = local read "Dp_error_d"() -> (w619:fxp<+/-,33,8>)
    n309 = local read "Kv_p"() -> (w620:fxp<+/-,22,8>)
    n310 = local read "Bv_p"() -> (w618:fxp<+/-,22,8>)
    n311 = local read "Kv_y"() -> (w629:fxp<+/-,22,8>)
    n312 = local read "Bv_y"() -> (w627:fxp<+/-,22,8>)
    n313 = local read "Force_y"() -> (w622:fxp<+/-,32,10>)
    n314 = Multiply(x=w628, y=w629) -> (x*y=w624:fxp<+/-,55,16>)
    n315 = Multiply(x=w626, y=w627) -> (x*y=w625:fxp<+/-,58,24>)
    n316 = Multiply(x=w619, y=w620) -> (x*y=w615:fxp<+/-,55,16>)
    n317 = Multiply(x=w617, y=w618) -> (x*y=w616:fxp<+/-,58,24>)
    n318 = local read "Force_p"() -> (w613:fxp<+/-,32,10>)
    n319 = Add(x=w624, y=w625) -> (x+y=w623:fxp<+/-,63,24>)
    n320 = Add(x=w615, y=w616) -> (x+y=w614:fxp<+/-,63,24>)
    n321 = Subtract(x=w623, y=w622) -> (x-y=→"fyt_d":fxp<+/-,63,24>)
    n322 = Subtract(x=w614, y=w613) -> (x-y=→"fpt_d":fxp<+/-,63,24>)
  }
  n323 = while "Encoder_p" {
    shift-right: [w640] -> _
    shift-left: _ -> [w641]
    shift-right: [w642] -> _
    shift-left: _ -> [w643]
    shift-right: [w636] -> _
    shift-left: _ -> [w644]
    stop <- FALSE stop-if-true
    w633 = fxp<+/-,32,0> 0.0020454544574022293  # L*(18/22)/800
    n324 = xnode "FPGA I/O Node"() -> ("Mod4/DI0"=w638:bool, "Mod4/DI1"=w639:bool)  [unwired: 2 in, 2 out]
    n325 = call "encoder_sub.vi"("A_pre"=w641, "B_pre"=w643, "Encoder Position_pre"=w644, "A input"=w638, "Encoder Position Reset"="Encoder reset_p", "B input"=w639) -> ("A"=w640:bool, "B"=w642:bool, "Encoder Position (Counts)"=w636:i32)  [unwired: 19 in]
    "Encoder Position_p" <- w636
    n326 = To Fixed-Point(number=w636) -> (fixed-point=w635:fxp<+/-,32,32>)  [unwired: 1 in]
    n327 = xnode "High Throughput Multiply"("x"=w635, "y"=w633) -> ("x*y"=→"D_p(mm)":fxp<+/-,64,32>)
    n328 = xnode "High Throughput Multiply"("x"=w635, "y"=fxp<+/-,16,1> 0.125) -> ("x*y"=→"rad_p(NrTheta)":fxp<+/-,48,33>)
  }
  n329 = while "Omega_p(T method)" {
    shift-right: [w655] -> _
    shift-left: _ -> [w653]
    shift-right: [w648] -> _
    shift-left: _ -> [w654]
    shift-right: [w650] -> _
    shift-left: _ -> [w652]
    stop <- FALSE stop-if-true
    w647 = fxp<+/-,32,0> 0.2604353614151478  # L/2/pi*(18/22)
    n330 = local read "Encoder Position_p"() -> (w655:i32)
    n331 = call "Tick Count4"() -> ("Tick Count(Ticks)"=w651:u32)
    n332 = call "omega_sub_Encoder_800ppr.vi"("omega_pre"=w654, "ticks_m_pre"=w652, "ticks"=w651, "count_pre"=w653, "count"=w655) -> ("ticks_m"=w650:u32, "mt"=→"mt_omega_p":u32, "omega"=w648:fxp<+/-,20,9>)  [unwired: 4 in]
    "omega_p (rad/s)" <- w648
    n333 = xnode "High Throughput Multiply"("x"=w647, "y"=w648) -> ("x*y"=→"Dp_d (mm/s)":fxp<+/-,52,9>)
  }
  n334 = xnode "FPGA I/O Node"("error in"=w1, "Mod6/Stop"=TRUE) -> ()  [unwired: 1 in, 2 out]
